vi "Create_Simple_Var.vi"(4 "Value":T1=variant(string "")) -> (1 "Var":refnum<class "Var_Variant.lvclass">)   [LabVIEW 2021, in "Var_Variant.lvclass"]
uses:
  Var_Variant.lvclass
  Var_Variant.lvclass/Var_Variant.ctl
  Type.ctl
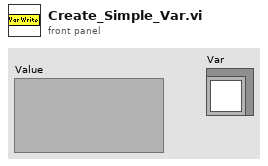
[diagram p1: front panel]
types:
  T1 = typedef "Var_Variant.lvclass/Type.ctl" = variant
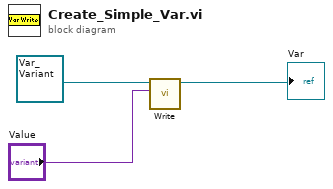
[diagram p0: block diagram]
diagram:
  n1 = call-dynamic "Write.vi"("Value"="Value", "Double Float.lvclass_340760 in"=refnum<class "Var_Variant.lvclass"> refnum ("Constants.lvlib:Numeric.lvclass")) -> ("Double Float.lvclass_340760 out"=→"Var":refnum<class "Var_Variant.lvclass">)  [unwired: 8 in, 1 out]
